vi "Actor Core.vi"(8 "error in":errorcluster, 11 "M_Butt in":refnum<class "Manual_Buttons.lvclass">) -> (0 "error out":errorcluster, 3 "Actor out":refnum<class "Actor.lvclass">)   [LabVIEW 2023, in "Manual_Buttons.lvlib" / "Manual_Buttons.lvclass"]
doc: "The user interface for this panel.\n\n----\nPlease see the following web address for additional documentation and tutorial information:\nhttp://www.mooregoodideas.com/mgi-panel-manager/\n\nAuthor: Derek Trepanier\n\nCopyright (c) 2018, Moore Good Ideas, Inc.\n\nAll rights reserved.\n\nRedistribution and use in source and binary forms, with or without modification, are permitted provided that the following conditions are met:\n\n * Redistributions of source code must retain the above copyright notice, this list of conditions and the following disclaimer.\n * Redistributions in binary form must reproduce the above copyright notice, this list of conditions and the following disclaimer in the documentation and/or other materials provided with the distribution.\n * Neither the name of Moore Good Ideas, Inc. nor the names of its contributors may be used to endorse or promote products derived from this software without specific prior written permission.\n\nTHIS SOFTWARE IS PROVIDED BY THE COPYRIGHT HOLDERS AND CONTRIBUTORS \"AS IS\" AND ANY EXPRESS OR IMPLIED WARRANTIES, INCLUDING, BUT NOT LIMITED TO, THE IMPLIED WARRANTIES OF MERCHANTABILITY AND FITNESS FOR A PARTICULAR PURPOSE ARE DISCLAIMED. IN NO EVENT SHALL THE COPYRIGHT OWNER OR CONTRIBUTORS BE LIABLE FOR ANY DIRECT, INDIRECT, INCIDENTAL, SPECIAL, EXEMPLARY, OR CONSEQUENTIAL DAMAGES (INCLUDING, BUT NOT LIMITED TO, PROCUREMENT OF SUBSTITUTE GOODS OR SERVICES; LOSS OF USE, DATA, OR PROFITS; OR BUSINESS INTERRUPTION) HOWEVER CAUSED AND ON ANY THEORY OF LIABILITY, WHETHER IN CONTRACT, STRICT LIABILITY, OR TORT (INCLUDING NEGLIGENCE OR OTHERWISE) ARISING IN ANY WAY OUT OF THE USE OF THIS SOFTWARE, EVEN IF ADVISED OF THE POSSIBILITY OF SUCH DAMAGE."
uses:
  Project/Manual_Buttons.lvclass
  C:/Users/Public/Documents/Development/builds/Engine/Engine.lvlibp/Project/Engine.lvclass
  builds/Engine/Actor Framework.lvlibp/1abvi3w/vi.lib/ActorFramework/Actor/Actor.lvclass
  M_Butt Messages/User Comment Dialog Msg/User Comment Dialog Msg.lvclass/User Comment Dialog Msg.ctl
  builds/Engine/Actor Framework.lvlibp/1abvi3w/vi.lib/ActorFramework/Message Enqueuer/Enqueue.vi
  builds/Engine/Engine.lvlibp/Accessors/Read Caller Q.vi
  M_Butt Messages/User Comment Dialog Msg/User Comment Dialog Msg.lvclass
  M_Butt Messages/New Test Name Dialog Msg/New Test Name Dialog Msg.lvclass
  M_Butt Messages/New Report Action Msg/New Report Action Msg.lvclass
  builds/Engine/Actor Framework.lvlibp/1abvi3w/vi.lib/ActorFramework/Message Enqueuer/Message Enqueuer.lvclass
  builds/Base Software/Panels/Right Panel.lvlibp/Project/Right.lvclass
  builds/Engine/Panel Manager.lvlibp/Panel Actor/Panel Actor.lvclass
  builds/Engine/Engine.lvlibp/Engine Messages/Reset Manual Layout Msg/Reset Manual Layout Msg.lvclass
  builds/Engine/Engine.lvlibp/Project/Engine.lvclass
  C:/Users/Public/Documents/Development/builds/Engine/Panel Manager.lvlibp/Panel Actor/Panel Actor.lvclass
panel:
  in  "Reset":bool
  in  "Comment":bool
  in  "New Test Name":bool
  in  "Live Report":bool
  in  "New Log":bool
  in  "Safe BTE":bool
  in  "Toggle Supplies":bool
  in  "Quick Start":bool
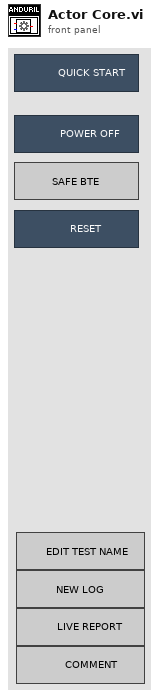
[diagram p1: front panel]
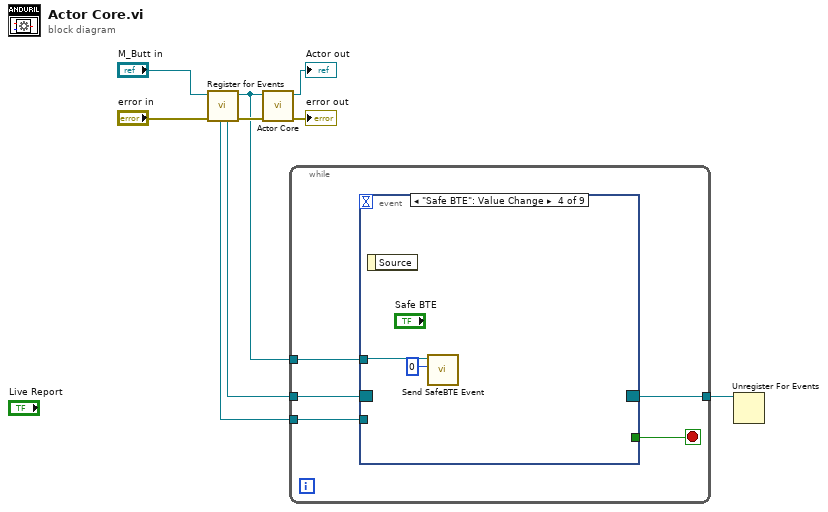
[diagram p0: block diagram]
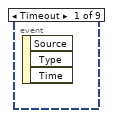
[diagram p2: hidden frame]
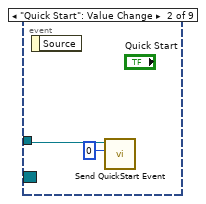
[diagram p3: hidden frame]
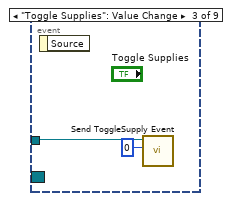
[diagram p4: hidden frame]
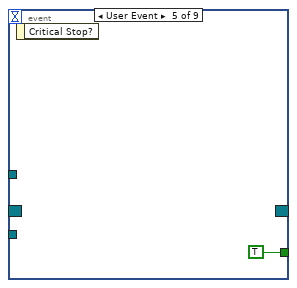
[diagram p5: hidden frame]
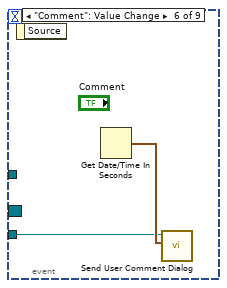
[diagram p6: hidden frame]
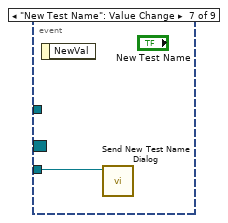
[diagram p7: hidden frame]
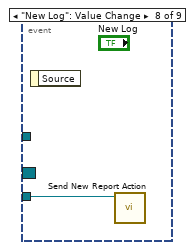
[diagram p8: hidden frame]
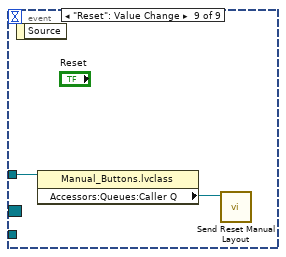
[diagram p9: hidden frame]
diagram:
  n1 = call "Register for Events.vi"("Error In"="error in", "Panel Actor in"="M_Butt in") -> ("Error Out"=w5:errorcluster, "Panel Actor out"=w2:refnum<class "Manual_Buttons.lvclass">, "Pnl Actor"=w4:refnum<event-registration>, "Self Enqueuer"=w1:refnum<class "Message Enqueuer.lvclass">)  [unwired: 6 in]
  n2 = call-parent "Actor Core.vi"("error in"=w5, "Right Panel in"=w2) -> ("error out"=→"error out":errorcluster, "Actor out"=→"Actor out":refnum<class "Actor.lvclass">)  [unwired: 8 in]
  n3 = while {
    tunnel: w4 -> [w14]
    tunnel: [w12] -> w3
    tunnel: w2 -> [w11]
    tunnel: w1 -> [w10]
    stop <- w13 stop-if-true
    n4 = event shown="[3] \"Safe BTE\": Value Change" {
      selector: w14 -> [_ _ _ _ _ _ _ _ _]
      dyn-events: [_ _ _ _ _ _ _ _ _] -> w12
      timeout: _ -> [_ _ _ _ _ _ _ _ _]
      tunnel: [_ _ _ _ TRUE _ _ _ _] -> w13
      tunnel: w11 -> [_ w16 w18 w20 _ _ _ _ w26]
      tunnel: w10 -> [_ _ _ _ _ w22 w24 w25 _]
      event Timeout {
        n5 = event-data() -> ()  [unwired: 1 in, 3 out]
      }
      event "Quick Start": Value Change {
        n6 = event-data() -> ()  [unwired: 1 in, 1 out]
        n7 = call "Send QuickStart Event.vi"("QuickStart"=0, "Engine in"=w16) -> ()  [unwired: 8 in, 2 out]
      }
      event "Toggle Supplies": Value Change {
        n8 = event-data() -> ()  [unwired: 1 in, 1 out]
        n9 = call "Send ToggleSupply Event.vi"("ToggleSupply"=0, "Engine in"=w18) -> ()  [unwired: 8 in, 2 out]
      }
      event "Safe BTE": Value Change {
        n10 = event-data() -> ()  [unwired: 1 in, 1 out]
        n11 = call "Send SafeBTE Event.vi"("SafeBTE"=0, "Engine in"=w20) -> ()  [unwired: 8 in, 2 out]
      }
      event User Event {
        n12 = event-data() -> ()  [unwired: 1 in, 1 out]
      }
      event "Comment": Value Change {
        n13 = event-data() -> ()  [unwired: 1 in, 1 out]
        n14 = Get Date/Time In Seconds() -> (seconds since 1Jan1904=w23:timestamp)
        n15 = call "Send User Comment Dialog.vi"("Timestamp"=w23, "Message Enqueuer"=w22) -> ()  [unwired: 8 in, 2 out]
      }
      event "New Test Name": Value Change {
        n16 = event-data() -> ()  [unwired: 1 in, 1 out]
        n17 = call "Send New Test Name Dialog.vi"("Message Enqueuer"=w24) -> ()  [unwired: 9 in, 2 out]
      }
      event "New Log": Value Change {
        n18 = event-data() -> ()  [unwired: 1 in, 1 out]
        n19 = call "Send New Report Action.vi"("Message Enqueuer"=w25) -> ()  [unwired: 9 in, 2 out]
      }
      event "Reset": Value Change {
        n20 = event-data() -> ()  [unwired: 1 in, 1 out]
        n21 = property class="Manual_Buttons.lvclass"(reference=w26) -> ("Accessors:Queues:Caller Q"=w27:refnum<class "Message Enqueuer.lvclass">)  [unwired: 1 in, 2 out]
        n22 = call "Send Reset Manual Layout.vi"("Message Enqueuer"=w27) -> ()  [unwired: 9 in, 2 out]
      }
    }
  }
  n23 = Unregister For Events(event registration refnum=w3) -> ()  [unwired: 1 in, 1 out]
